vi "AMview.vi"() -> ()   [LabVIEW 2014]
uses:
  TypeDefs/Color.ctl
  TypeDefs/CameraEvent.ctl
  TypeDefs/Camera.ctl
  <vilib>/Utility/miscctls.llb/LV3DPointTypeDef.ctl
  <vilib>/Utility/miscctls.llb/LVStringsAndValuesArrayTypeDef_U16.ctl
  TypeDefs/Point3D.ctl
  <vilib>/picture/3D Picture Control/Object/Add Object (no reference).vi
  <vilib>/picture/3D Picture Control/Object/Create Object (name).vi
  <vilib>/xml/Close Reference(Node).vi
  <vilib>/picture/3D Picture Control/NI_3D Picture Control.lvlib
  <vilib>/xml/NI_XML.lvlib
  <resource>/objmgr/DOMUserDefRef.rc
panel:
  in  "stop":bool
  in  "Toolbar":T1(tab)
  in  "Load":bool
  in  "Line Width":dbl=1.0
  in  "Color Off":T2={"Alpha"=1.0, "Color"=0} {"Alpha" min=0.0 max=1.0 scale=0.0..1.0}
  in  "Line Color":u32(colorbox)=6618880
  in  "Reset":bool
  in  "Ports":enum16{"One Viewport", "Four Viewports"}(ring)
  in  "Build Plate Color":u32(colorbox)=6618880
  in  "Color On":T2={"Alpha"=1.0, "Color"=0} {"Alpha" min=0.0 max=1.0 scale=0.0..1.0}
  in  "Scale":bool
  in  "Percent":dbl=50.0 min=1.0 max=200.0
  in  "ZT":dbl=1.0
  in  "ZPT":bool
  in  "ZNT":bool
  in  "YT":dbl=1.0
  in  "YPT":bool
  in  "YNT":bool
  in  "XT":dbl=1.0
  in  "XPT":bool
  in  "XNT":bool
  in  "Zcen":dbl
  in  "Ycen":dbl
  in  "Xcen":dbl
  in  "Zmax":dbl
  in  "Zmin":dbl
  in  "Ymax":dbl
  in  "Ymin":dbl
  in  "Xmax":dbl
  in  "Xmin":dbl
  in  "ZR":dbl=90.0
  in  "ZRR":bool
  in  "ZLR":bool
  in  "YR":dbl=90.0
  in  "YRR":bool
  in  "YLR":bool
  in  "XR":dbl=90.0
  in  "XRR":bool
  in  "XLR":bool
  in  "Model Selector":u16(ring) items=["GE_SnapBlock_18x9_Repaired"]
  in  "Model Color":T2={"Alpha"=1.0, "Color"=0} {"Alpha" min=0.0 max=1.0 scale=0.0..1.0}
  in  "Layer Thickness":dbl=1.0
  in  "Beam Size":dbl=1.0
  in  "Build Size":dbl=100.0
  in  "SavePath":bool
  in  "Slice":bool
  in  "Z":dbl
  in  "SaveXML":bool
  in  "GenLayer":bool
  out "XML":string
  # "X-->"
  # "Translation"
  # "Scale/Sym"
  # "Rotation"
  # "Bounds"
  # "Y-->"
  # "Z-->"
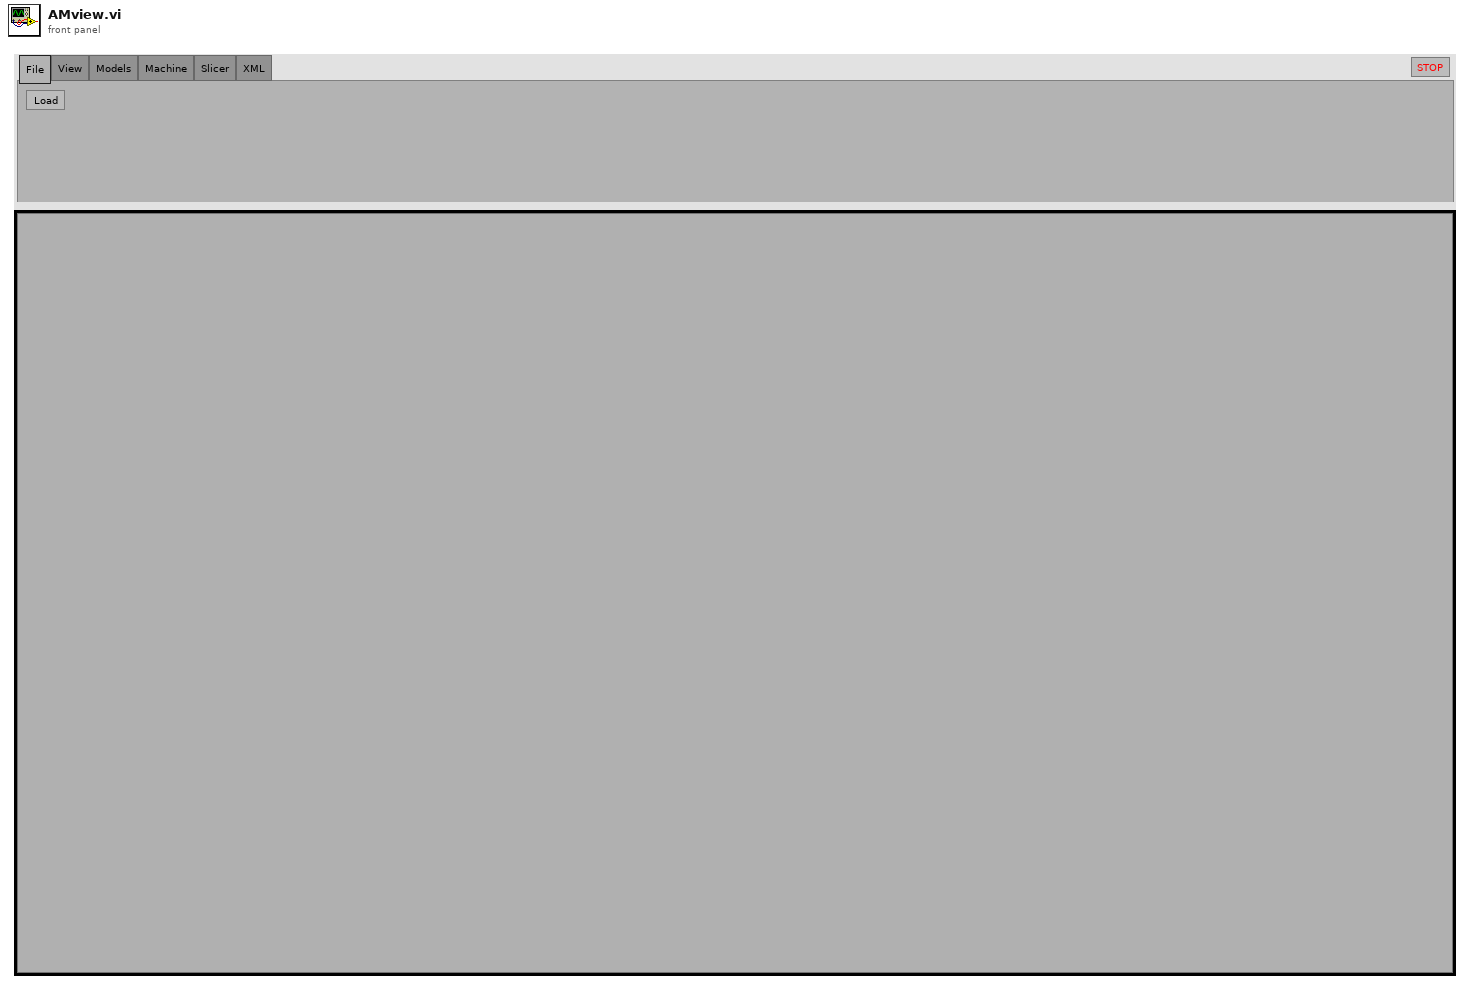
[diagram p1: front panel]
types:
  T1 = enum32{"File", "View", "Models", "Machine", "Slicer", "XML"}
  T2 = typedef "Color.ctl" = cluster{"Alpha":dbl, "Color":u32}
  T3 = enum16{"Add", "Get", "Scale", "Rotate", "Translate", "Symmetry", "Clear"}
  T4 = enum16{"New", "Find", "FindPattern", "GetTable", "Clear"}
  T5 = typedef "LVStringsAndValuesArrayTypeDef_U16.ctl" = cluster{"String":string, "Value":u16}[]
  T6 = typedef "CameraEvent.ctl" = cluster{"Camera":T7, "Task":enum16{"redraw", "setTo", "setToUpdate"}}
  T7 = typedef "Camera.ctl" = cluster{"Camera Position":T8, "Target":T8, "Up Direction":T8}
  T8 = typedef "LV3DPointTypeDef.ctl" = cluster{"X":sgl, "Y":sgl, "Z":sgl}
  T9 = enum16{"Add", "Get", "Scale", "Rotate", "Translate", "Symmetry"}
  T10 = enum16{"Overall", "Per Primitive", "Per Vertex", "Binding Off"}
  T11 = enum16{"Points", "Lines", "Line Strip", "Line Loop", "Triangles", "Triangle Strip", "Triangle Fan", "Quads", "Quad Strip", "Polygon"}
  T12 = cluster{"Axis":enum16{"X", "Y", "Z"}, "Angle":sgl}
  T13 = typedef "Point3D.ctl" = cluster{"X":sgl, "Y":sgl, "Z":sgl}
  T14 = typedef "TriangleFace.ctl" = cluster{"Normal":T13, "Vertex1":T13, "Vertex2":T13, "Vertex3":T13}
  T15 = typedef "Line2D.ctl" = cluster{"Vertex1":T16, "Vertex2":T16, "Slope":dbl}
  T16 = typedef "Point2DwSlope.ctl" = cluster{"X":sgl, "Y":sgl, "Slope":dbl}
  T17 = typedef "Poly2DwSlope.ctl" = cluster{"VertexArray":T16[]}
  T18 = cluster{"VertexArray":T16[], "OnOffAr":enum16{"On", "Off"}[]}
  T19 = cluster{"VertexArray":T16[], enum16{"On", "Off"}[]}
  T20 = cluster{"VertexArray":T16[], "OnOffAr":enum16{"On", "Off"}[]}[]
  T21 = typedef "XYonOffArray.ctl" = cluster{"X":dbl, "Y":dbl, "OnOff":bool}[]
  T22 = typedef "LVRGBAColorTypeDef.ctl" = cluster{"Red":sgl, "Green":sgl, "Blue":sgl, "Alpha":sgl}
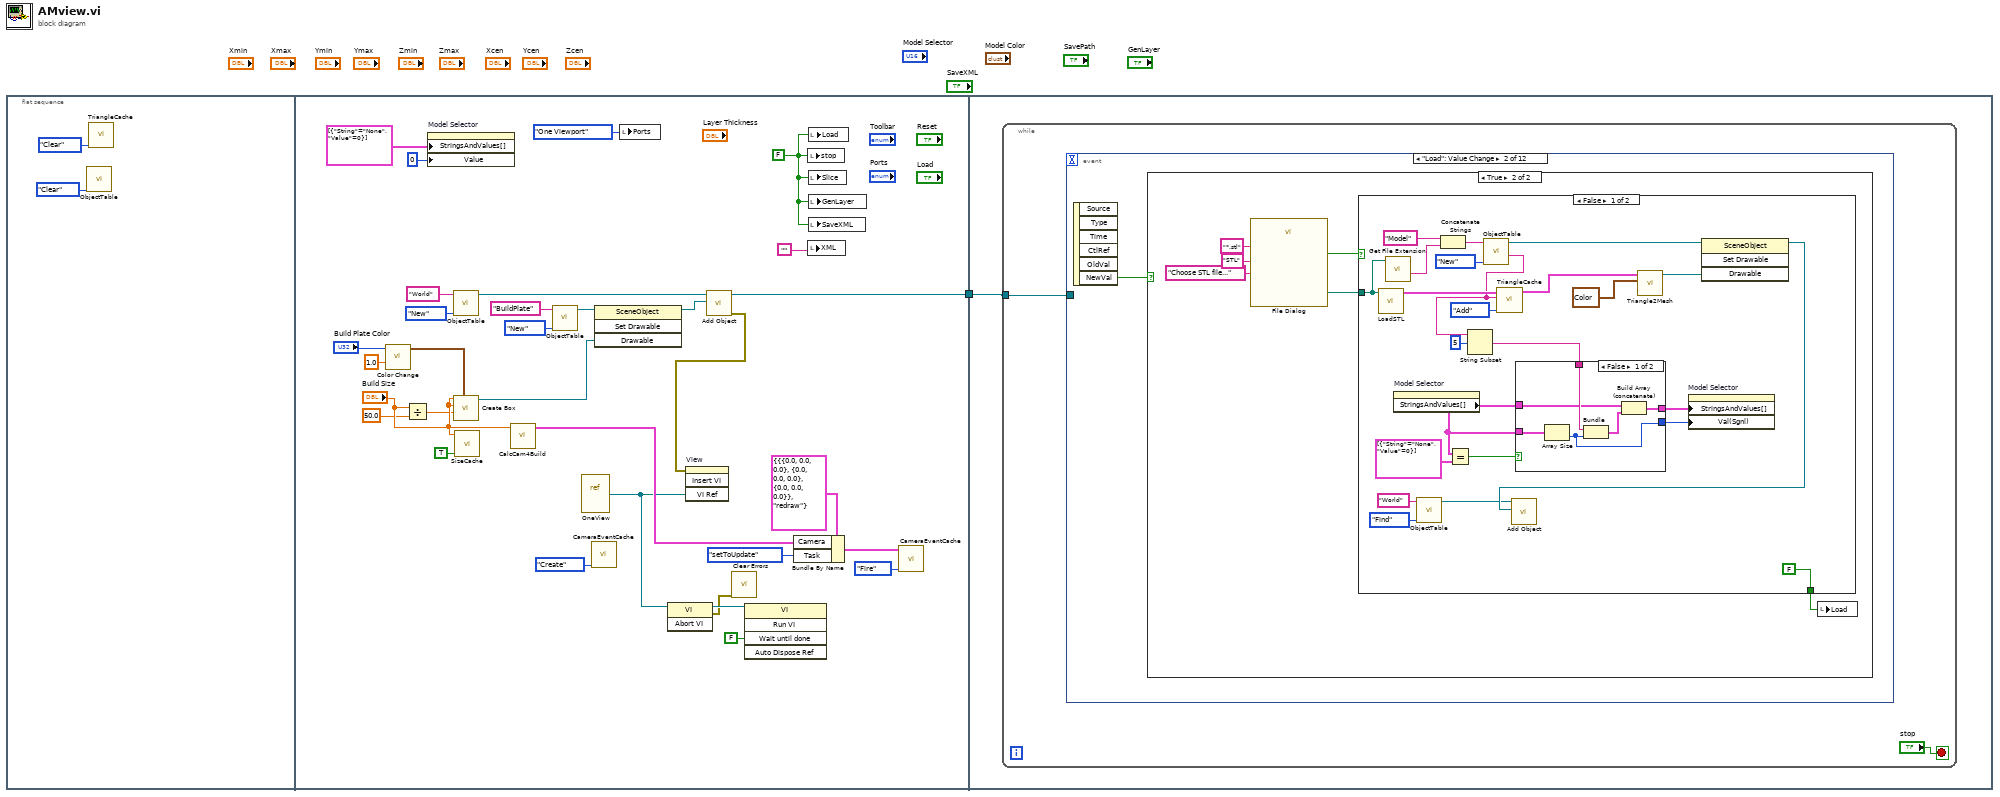
[diagram p0: block diagram]
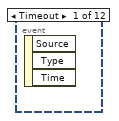
[diagram p2: hidden frame]
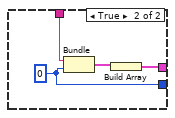
[diagram p4: hidden frame]
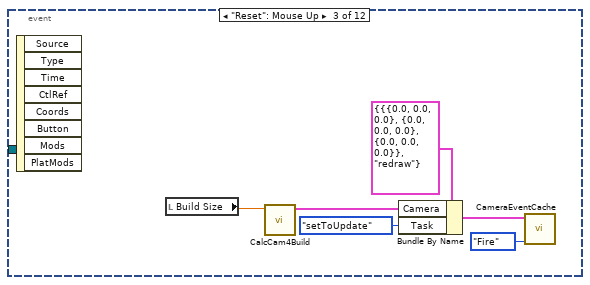
[diagram p6: hidden frame]
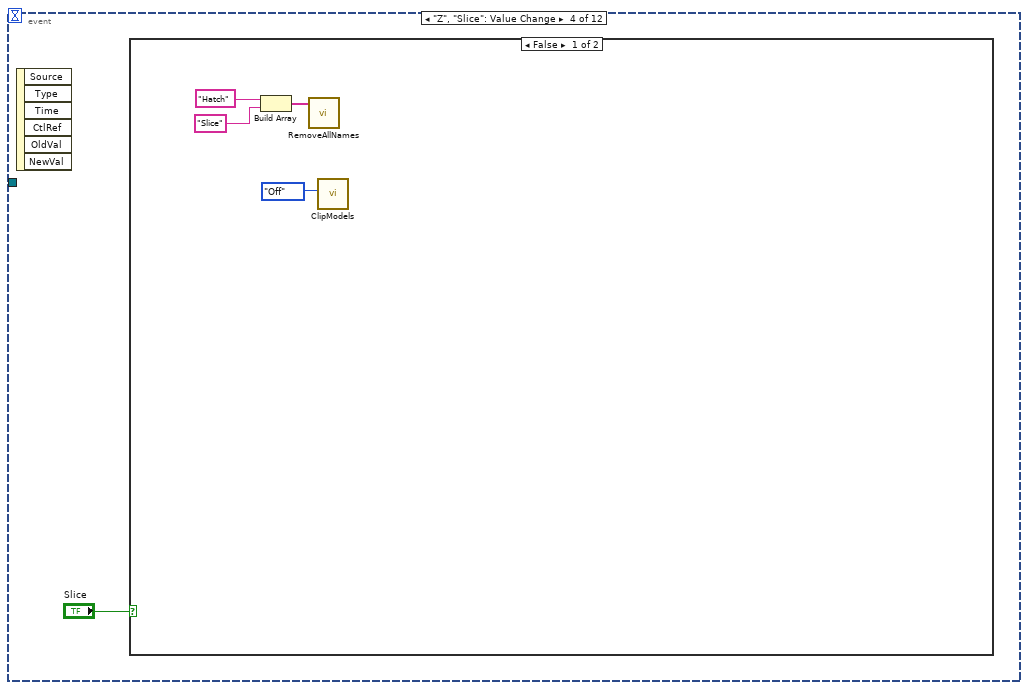
[diagram p7: hidden frame]
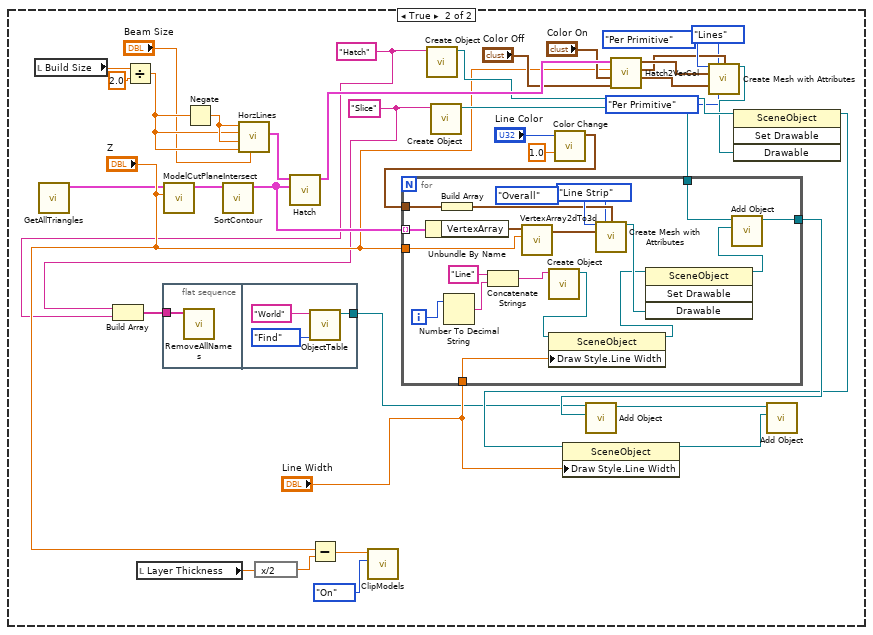
[diagram p8: hidden frame]
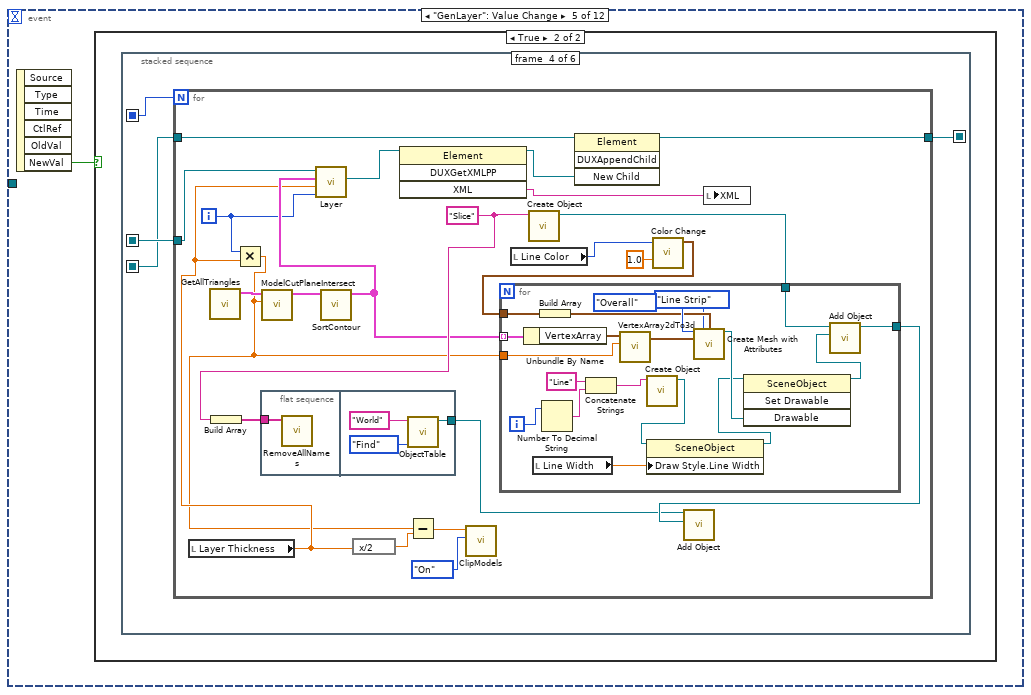
[diagram p9: hidden frame]
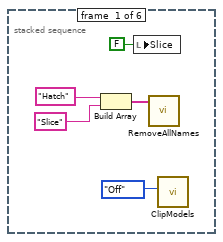
[diagram p11: hidden frame]
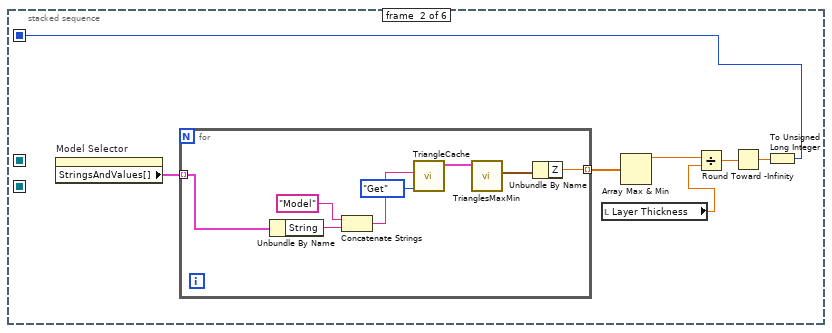
[diagram p12: hidden frame]
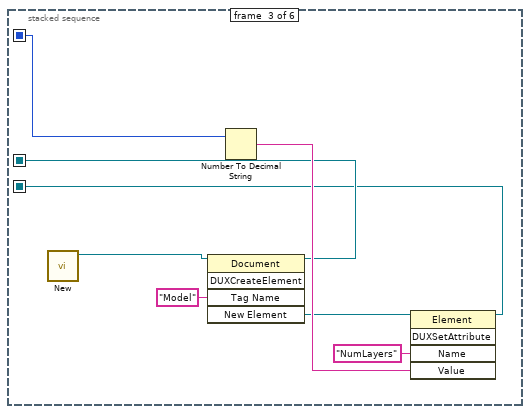
[diagram p13: hidden frame]
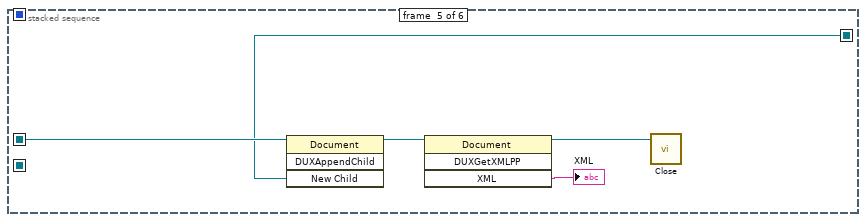
[diagram p14: hidden frame]
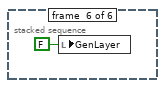
[diagram p15: hidden frame]
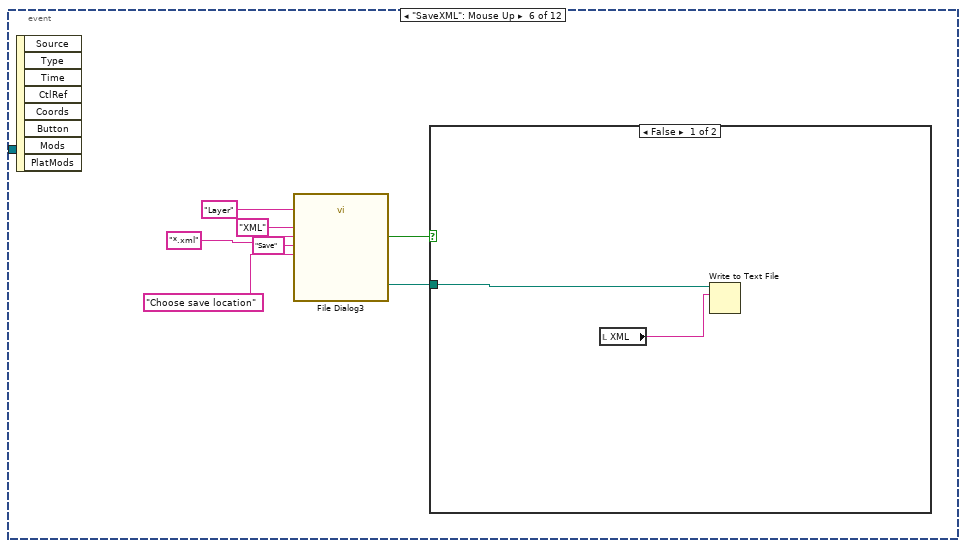
[diagram p16: hidden frame]
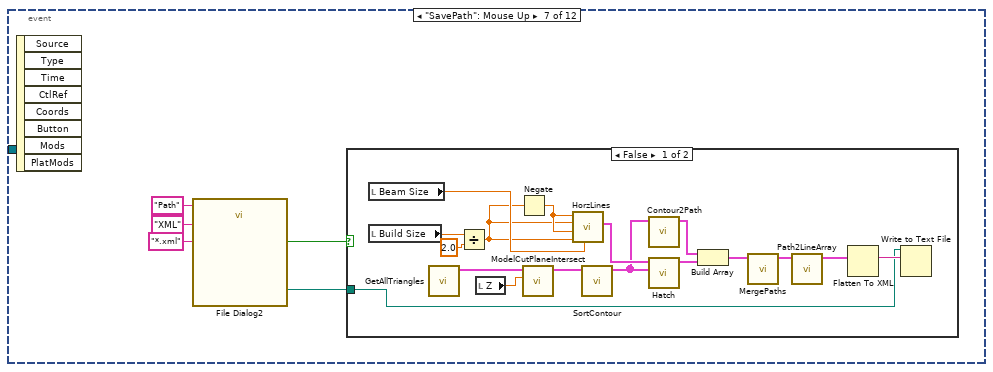
[diagram p18: hidden frame]
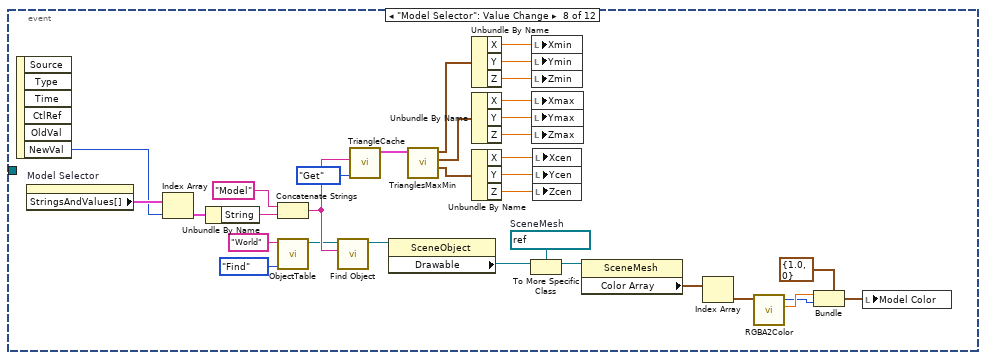
[diagram p20: hidden frame]
diagram:
  n1 = flat-sequence {
    tunnel: [w13] -> w1
    tunnel: w1 -> [w36]
    frame #0 {
      n2 = call "ObjectTable.vi"("ObjectStoreSelector"=T4."Clear") -> ()  [unwired: 6 in, 5 out]
      n3 = call "TriangleCache.vi"("TriangleOperations"=T3."Clear") -> ()  [unwired: 10 in, 1 out]
    }
    frame #1 {
      w5 = FALSE ("stop")
      n4 = call <vilib>:"Color Change.vi"("Alpha"=1.0, "Color"="Build Plate Color") -> ("RGBA"=w17:cluster{"R":sgl, "G":sgl, "B":sgl, "A":sgl})  [unwired: 9 in]
      n5 = Divide(x="Build Size", y=50.0) -> (x/y=w15:dbl)
      n6 = property on="Model Selector" class="Ring (strict)"("StringsAndValues[]"=T5 [{"String"="None", "Value"=0}] ("Strings And Values []"), "Value"=0) -> ()  [unwired: 2 in, 2 out]
      n7 = call "ObjectTable.vi"("ObjectStoreSelector"=enum16{"New", "Find", "FindPattern", "GetTable"}."New", "Name"="World") -> ("ObjectRef"=w31:refnum<vi>)  [unwired: 5 in, 4 out]
      n8 = call <vilib>:"Create Box.vi"("Color"=w17, "Length Z"=w15, "Length Y"="Build Size", "Length X"="Build Size") -> ("New Box Refnum"=w19:refnum<vi>)  [unwired: 6 in, 1 out]
      n9 = call "SizeCache.vi"("Set"=TRUE, "SizeIn"="Build Size") -> ()  [unwired: 9 in, 1 out]
      n10 = call "CalcCam4Build.vi"("BuildSize"="Build Size") -> ("CamOut"=w25:T7)  [unwired: 10 in]
      n11 = call "ObjectTable.vi"("ObjectStoreSelector"=enum16{"New", "Find", "FindPattern", "GetTable"}."New", "Name"="BuildPlate") -> ("ObjectRef"=w33:refnum<vi>)  [unwired: 5 in, 4 out]
      n12 = vi-ref "OneView.vi"() -> (w9:refnum<vi>)
      n13 = call "CameraEventCache.vi"("Operation"=enum16{"Create", "GetRef", "Fire"}."Create") -> ()  [unwired: 10 in, 1 out]
      n14 = invoke class="SceneObject" method="Set Drawable"(reference=w33, "Drawable"=w19) -> (reference out=w20:refnum<vi>)  [unwired: 2 in, 3 out]
      n15 = local write "Ports"(enum16{"One Viewport", "Four Viewports"}."One Viewport" ("Ports")) -> ()
      n16 = invoke class="VI" method="Abort VI"(reference=w9) -> (reference out=w10:refnum<vi>, error out=w6:errorcluster)  [unwired: 2 in, 1 out]
      n17 = call-poly <vilib>:"Add Object.vi"("New Object In"=w20, "Scene Object In"=w31) -> ("error out"=w35:errorcluster, "Scene Object Out"=w13:refnum<vi>)  [unwired: 8 in]
      n18 = invoke on="View" class="SubPanel" method="Insert VI"(error in=w35, "VI Ref"=w9) -> ()  [unwired: 2 in, 4 out]
      n19 = call <vilib>:"Clear Errors.vi"("error in (no error)"=w6) -> ()  [unwired: 5 in, 2 out]
      n20 = invoke class="VI" method="Run VI"(reference=w10, "Wait until done"=FALSE ("Wait Until Done")) -> ()  [unwired: 3 in, 5 out]
      n21 = Bundle By Name(cluster=T6 {"Camera"={"Camera Position"={"X"=0.0, "Y"=0.0, "Z"=0.0}, "Target"={"X"=0.0, "Y"=0.0, "Z"=0.0}, "Up Direction"={"X"=0.0, "Y"=0.0, "Z"=0.0}}, "Task"=enum."redraw"} ("CameraEvent"), "Camera"=w25, "Task"=enum16{"redraw", "setTo", "setToUpdate"}."setToUpdate") -> (w24:T6)
      n22 = local write "stop"(w5) -> ()
      n23 = local write "XML"("") -> ()
      n24 = local write "Load"(w5) -> ()
      n25 = local write "Slice"(w5) -> ()
      n26 = local write "GenLayer"(w5) -> ()
      n27 = local write "SaveXML"(w5) -> ()
      n28 = call "CameraEventCache.vi"("Operation"=enum16{"Create", "GetRef", "Fire"}."Fire", "CameraEvent"=w24) -> ()  [unwired: 9 in, 1 out]
    }
    frame #2 {
      n29 = while {
        tunnel: w36 -> [w37]
        stop <- "stop" stop-if-true
        n30 = event shown="[1] \"Load\": Value Change" {
          selector: _ -> [_ _ _ _ _ _ _ _ _ _ _ _]
          dyn-events: _ -> [_ _ _ _ _ _ _ _ _ _ _ _]
          timeout: _ -> [_ _ _ _ _ _ _ _ _ _ _ _]
          tunnel: w37 -> [_ _ _ _ _ _ _ _ _ _ _ _]
          event Timeout {
            n31 = event-data() -> ()  [unwired: 1 in, 3 out]
          }
          event "Load": Value Change {
            n32 = event-data() -> ("NewVal"=w39:bool)  [unwired: 1 in, 5 out]
            n33 = case shown="True" w39 {
              frame False {
              }
              frame True {
                n34 = call "File Dialog"("prompt"="Choose STL file...", "pattern (all files)"="*.stl", "pattern label"="STL") -> ("selected path"=w41:path, "cancelled"=w42:bool)  [unwired: 9 in, 2 out]
                n35 = case shown="False" w42 {
                  tunnel: w41 -> [w54 _]
                  tunnel: [FALSE _] -> w40
                  frame False {
                    n36 = call "LoadSTL.vi"("STL Path"=w54) -> ("Triangles"=w59:T14[])  [unwired: 8 in, 2 out]
                    n37 = call <vilib>:"Get File Extension.vi"("file"=w54) -> ("filename without extension"=w53:string)  [unwired: 7 in, 3 out]
                    n38 = property on="Model Selector" class="Ring (strict)"() -> ("StringsAndValues[]"=w48:T5)  [unwired: 2 in, 2 out]
                    n39 = call "ObjectTable.vi"("ObjectStoreSelector"=enum16{"New", "Find", "FindPattern", "GetTable"}."Find", "Name"="World") -> ("ObjectRef"=w63:refnum<vi>)  [unwired: 5 in, 4 out]
                    n40 = Concatenate Strings("Model" ("Name"), w53) -> (w66:string)
                    n41 = Equal?(x=w48, y=T5 [{"String"="None", "Value"=0}] ("Strings And Values []")) -> (x = y?=w47:bool)
                    n42 = call "ObjectTable.vi"("ObjectStoreSelector"=enum16{"New", "Find", "FindPattern", "GetTable"}."New", "Name"=w66) -> ("UniqueName"=w51:string, "ObjectRef"=w64:refnum<vi>)  [unwired: 5 in, 3 out]
                    n43 = String Subset(string=w51, offset (0)=5) -> (substring=w52:string)  [unwired: 1 in]
                    n44 = call "TriangleCache.vi"("TriangleOperations"=T9."Add", "ModelName"=w51, "TrianglesIn"=w59) -> ("TrianglesOut"=w58:T14[])  [unwired: 8 in]
                    n45 = case shown="False" w47 {
                      tunnel: [w74 w77] -> w56
                      tunnel: [w73 w76] -> w55
                      tunnel: w52 -> [w72 w79]
                      tunnel: w48 -> [w71 _]
                      tunnel: w48 -> [w70 _]
                      frame False {
                        n46 = Array Size(array=w70) -> (size(s)=w73:i32)
                        n47 = Bundle("UniqueName"=w72, w73) -> (w75:cluster{"UniqueName":string, i32})  [unwired: 1 in]
                        n48 = Build Array (concatenate)(w71, w75) -> (w74:cluster{"UniqueName":string, "Value":i32}[])
                      }
                      frame True {
                        w76 = 0
                        n49 = Bundle("UniqueName"=w79, w76) -> (w78:cluster{"UniqueName":string, i32})  [unwired: 1 in]
                        n50 = Build Array(w78) -> (w77:cluster{"UniqueName":string, i32}[])
                      }
                    }
                    n51 = call "Triangle2Mesh.vi"("Color"=T2 {"Alpha"=1.0, "Color"=16711680}, "Triangles"=w58) -> ("Refnum"=w60:refnum<vi>)  [unwired: 9 in]
                    n52 = property on="Model Selector" class="Ring (strict)"("StringsAndValues[]"=w56, "Val(Sgnl)"=w55) -> ()  [unwired: 2 in, 2 out]
                    n53 = invoke class="SceneObject" method="Set Drawable"(reference=w64, "Drawable"=w60) -> (reference out=w69:refnum<vi>)  [unwired: 2 in, 3 out]
                    n54 = call-poly <vilib>:"Add Object.vi"("New Object In"=w69, "Scene Object In"=w63) -> ()  [unwired: 8 in, 2 out]
                  }
                  frame True {
                  }
                }
                n55 = local write "Load"(w40) -> ()
              }
            }
          }
          event "Reset": Mouse Up {
            n56 = event-data() -> ()  [unwired: 1 in, 8 out]
            n57 = local read "Build Size"() -> (w82:dbl)
            n58 = call "CalcCam4Build.vi"("BuildSize"=w82) -> ("CamOut"=w83:T7)  [unwired: 10 in]
            n59 = Bundle By Name(cluster=T6 {"Camera"={"Camera Position"={"X"=0.0, "Y"=0.0, "Z"=0.0}, "Target"={"X"=0.0, "Y"=0.0, "Z"=0.0}, "Up Direction"={"X"=0.0, "Y"=0.0, "Z"=0.0}}, "Task"=enum."redraw"} ("CameraEvent"), "Camera"=w83, "Task"=enum16{"redraw", "setTo", "setToUpdate"}."setToUpdate") -> (w81:T6)
            n60 = call "CameraEventCache.vi"("Operation"=enum16{"Create", "GetRef", "Fire"}."Fire", "CameraEvent"=w81) -> ()  [unwired: 9 in, 1 out]
          }
          event "Z", "Slice": Value Change {
            n61 = event-data() -> ()  [unwired: 1 in, 6 out]
            n62 = case shown="False" "Slice" {
              frame False {
                n63 = Build Array("Hatch", "Slice") -> (w89:string[])
                n64 = call "RemoveAllNames.vi"("Names"=w89) -> ()  [unwired: 11 in]
                n65 = call "ClipModels.vi"("Clip Plane State"=enum16{"Inherit Value", "Off", "On"}."Off") -> ()  [unwired: 11 in]
              }
              frame True {
                w93 = "Hatch" ("Name")
                w94 = "Slice" ("Name")
                n66 = local read "Build Size"() -> (w126:dbl)
                n67 = call "GetAllTriangles.vi"() -> ("AllTriangles"=w97:T14[])  [unwired: 11 in]
                n68 = Build Array(w94, w93) -> (w92:string[])
                n69 = Divide(x=w126, y=2.0) -> (x/y=w123:dbl)
                n70 = local read "Layer Thickness"() -> (w99:dbl)
                n71 = flat-sequence {
                  tunnel: w92 -> [w129]
                  tunnel: [w130] -> w91
                  frame #0 {
                    n72 = call "RemoveAllNames.vi"("Names"=w129) -> ()  [unwired: 11 in]
                  }
                  frame #1 {
                    n73 = call "ObjectTable.vi"("ObjectStoreSelector"=T4."Find", "Name"="World") -> ("ObjectRef"=w130:refnum<vi>)  [unwired: 5 in, 4 out]
                  }
                }
                n74 = call "ModelCutPlaneIntersect.vi"("CuttingZ"="Z", "Triangles"=w97) -> ("LineArray"=w128:T15[])  [unwired: 8 in, 1 out]
                n75 = Negate(x=w123) -> (-x=w124:dbl)
                n76 = call "SortContour.vi"("LineArray"=w128) -> ("Polys"=w122:T17[])  [unwired: 10 in]
                n77 = call "HorzLines.vi"("Spacing"="Beam Size", "yMax"=w123, "yMin"=w124, "xMax"=w123, "xMin"=w124) -> ("Poly2D"=w127:T17)  [unwired: 5 in, 1 out]
                n78 = expression code="x/2"(w99) -> (w98:dbl)
                n79 = call "Hatch.vi"("Polys"=w122, "Hatch"=w127) -> ("Path"=w116:T18)  [unwired: 9 in]
                n80 = Subtract(x="Z", y=w98) -> (x-y=w96:dbl)
                n81 = call "ClipModels.vi"("Clip Plane State"=enum16{"Inherit Value", "Off", "On"}."On", "Z"=w96) -> ()  [unwired: 10 in]
                n82 = call-poly <vilib>:"Create Object.vi"("Name"=w93) -> ("Scene:New Object"=w109:refnum<vi>)  [unwired: 9 in, 1 out]
                n83 = call-poly <vilib>:"Create Object.vi"("Name"=w94) -> ("Scene:New Object"=w119:refnum<vi>)  [unwired: 9 in, 1 out]
                n84 = call <vilib>:"Color Change.vi"("Alpha"=1.0, "Color"="Line Color") -> ("RGBA"=w120:cluster{"R":sgl, "G":sgl, "B":sgl, "A":sgl})  [unwired: 9 in]
                n85 = for {
                  tunnel: w122 -> [w150] mode=indexing
                  tunnel: "Z" -> [w148]
                  tunnel: w120 -> [w146]
                  tunnel: w119 -> [w139]
                  tunnel: [w138] -> w118
                  tunnel: "Line Width" -> [w133]
                  i -> [w142]
                  n86 = Unbundle By Name(w150) -> ("VertexArray"=w149:T16[])
                  n87 = Build Array(w146) -> (w145:cluster{"R":sgl, "G":sgl, "B":sgl, "A":sgl}[])
                  n88 = Number To Decimal String(number=w142) -> (decimal integer string=w141:string)  [unwired: 1 in]
                  n89 = Concatenate Strings("Line" ("string"), w141) -> (w140:string)
                  n90 = call "VertexArray2dTo3d.vi"("Z"=w148, "VertexArray2D"=w149) -> ("VertexArray3D"=w147:T13[])  [unwired: 9 in]
                  n91 = call-poly <vilib>:"Create Object.vi"("Name"=w140) -> ("Scene:New Object"=w135:refnum<vi>)  [unwired: 9 in, 1 out]
                  n92 = property class="SceneObject"(reference=w135, "Draw Style.Line Width"=w133) -> (reference out=w134:refnum<vi>)  [unwired: 1 in, 1 out]
                  n93 = call <vilib>:"Create Mesh with Attributes.vi"("Draw Mode"=T11."Line Strip", "Color Binding Mode"=T10."Overall", "Color Array"=w145, "Vertex Array"=w147) -> ("New Mesh Refnum"=w137:refnum<vi>)  [unwired: 10 in, 1 out]
                  n94 = invoke class="SceneObject" method="Set Drawable"(reference=w134, "Drawable"=w137) -> (reference out=w136:refnum<vi>)  [unwired: 2 in, 3 out]
                  n95 = call-poly <vilib>:"Add Object.vi"("New Object In"=w136, "Scene Object In"=w139) -> ("Scene Object Out"=w138:refnum<vi>)  [unwired: 8 in, 1 out]
                }
                n96 = call-poly <vilib>:"Add Object.vi"("New Object In"=w118, "Scene Object In"=w91) -> ("Scene Object Out"=w107:refnum<vi>)  [unwired: 8 in, 1 out]
                n97 = call "Hatch2VerCol.vi"("Color Off"="Color Off", "Color On"="Color On", "Z"="Z", "Path"=w116) -> ("Normals"=w102:T13[], "Colors"=w111:cluster{"R":sgl, "G":sgl, "B":sgl, "A":sgl}[], "VertexArray3d"=w112:T13[])  [unwired: 5 in]
                n98 = call <vilib>:"Create Mesh with Attributes.vi"("Draw Mode"=T11."Lines", "Color Binding Mode"=T10."Per Primitive", "Color Array"=w111, "Vertex Array"=w112, "Normal Array"=w102, "Normal Binding Mode"=T10."Per Primitive") -> ("New Mesh Refnum"=w108:refnum<vi>)  [unwired: 8 in, 1 out]
                n99 = invoke class="SceneObject" method="Set Drawable"(reference=w109, "Drawable"=w108) -> (reference out=w105:refnum<vi>)  [unwired: 2 in, 3 out]
                n100 = property class="SceneObject"(reference=w105, "Draw Style.Line Width"="Line Width") -> (reference out=w103:refnum<vi>)  [unwired: 1 in, 1 out]
                n101 = call-poly <vilib>:"Add Object.vi"("New Object In"=w103, "Scene Object In"=w107) -> ()  [unwired: 8 in, 2 out]
              }
            }
          }
          event "GenLayer": Value Change {
            n102 = event-data() -> ("NewVal"=w152:bool)  [unwired: 1 in, 5 out]
            n103 = case shown="True" w152 {
              frame False {
              }
              frame True {
                n104 = stacked-sequence {
                  seq-local: [_ w158 _ _ _ _] -> [_ _ w175 w184 _ _]
                  seq-local: [_ _ w174 _ _ _] -> [_ _ _ w183 w235 _]
                  seq-local: [_ _ w173 _ _ _] -> [_ _ _ w182 _ _]
                  seq-local: [_ _ _ w181 _ _] -> [_ _ _ _ w234 _]
                  frame #0 {
                    n105 = Build Array("Hatch", "Slice") -> (w155:string[])
                    n106 = local write "Slice"(FALSE ("Slice")) -> ()
                    n107 = call "RemoveAllNames.vi"("Names"=w155) -> ()  [unwired: 11 in]
                    n108 = call "ClipModels.vi"("Clip Plane State"=enum16{"Inherit Value", "Off", "On"}."Off") -> ()  [unwired: 11 in]
                  }
                  frame #1 {
                    n109 = property on="Model Selector" class="Ring (strict)"() -> ("StringsAndValues[]"=w164:T5)  [unwired: 2 in, 2 out]
                    n110 = for {
                      tunnel: w164 -> [w167] mode=indexing
                      tunnel: [w165] -> w163 mode=indexing
                      n111 = Unbundle By Name(w167) -> ("String"=w172:string)
                      n112 = Concatenate Strings("Model" ("string"), w172) -> (w168:string)
                      n113 = call "TriangleCache.vi"("TriangleOperations"=T3."Get", "ModelName"=w168) -> ("TrianglesOut"=w169:T14[])  [unwired: 9 in]
                      n114 = call "TrianglesMaxMin.vi"("Triangles"=w169) -> ("MaxDims"=w166:T13)  [unwired: 8 in, 2 out]
                      n115 = Unbundle By Name(w166) -> ("Z"=w165:sgl)
                    }
                    n116 = local read "Layer Thickness"() -> (w161:dbl)
                    n117 = Array Max & Min(array=w163) -> (max value=w162:sgl)  [unwired: 3 out]
                    n118 = Divide(x=w162, y=w161) -> (x/y=w160:dbl)
                    n119 = Round Toward -Infinity(1:w160) -> (0:w159:dbl)
                    n120 = To Unsigned Long Integer(number=w159) -> (unsigned 32bit integer=w158:u32)
                  }
                  frame #2 {
                    n121 = call <vilib>:"New.vi"() -> ("DOM document out"=w177:refnum<k20>)  [unwired: 8 in, 1 out]
                    n122 = invoke class="Document" method="DUXCreateElement"(reference=w177, "Tag Name"="Model") -> (reference out=w174:refnum<k20>, "New Element"=w176:refnum<k20>)  [unwired: 3 in, 3 out]
                    n123 = Number To Decimal String(number=w175) -> (decimal integer string=w178:string)  [unwired: 1 in]
                    n124 = invoke class="Element" method="DUXSetAttribute"(reference=w176, "Name"="NumLayers", "Value"=w178) -> (reference out=w173:refnum<k20>)  [unwired: 2 in, 4 out]
                  }
                  frame #3 {
                    n125 = for {
                      N: w184 -> [_]
                      tunnel: w183 -> [w194]
                      tunnel: w182 -> [w192]
                      tunnel: [w191] -> w181
                      i -> [w190]
                      w197 = "Slice" ("Name")
                      n126 = local read "Layer Thickness"() -> (w189:dbl)
                      n127 = call "GetAllTriangles.vi"() -> ("AllTriangles"=w200:T14[])  [unwired: 11 in]
                      n128 = Build Array(w197) -> (w196:string[])
                      n129 = Multiply(x=w190, y=w189) -> (x*y=w188:dbl)
                      n130 = flat-sequence {
                        tunnel: w196 -> [w208]
                        tunnel: [w209] -> w195
                        frame #0 {
                          n131 = call "RemoveAllNames.vi"("Names"=w208) -> ()  [unwired: 11 in]
                        }
                        frame #1 {
                          n132 = call "ObjectTable.vi"("ObjectStoreSelector"=T4."Find", "Name"="World") -> ("ObjectRef"=w209:refnum<vi>)  [unwired: 5 in, 4 out]
                        }
                      }
                      n133 = call "ModelCutPlaneIntersect.vi"("CuttingZ"=w188, "Triangles"=w200) -> ("LineArray"=w206:T15[])  [unwired: 8 in, 1 out]
                      n134 = call "SortContour.vi"("LineArray"=w206) -> ("Polys"=w193:T17[])  [unwired: 10 in]
                      n135 = call "Layer.vi"("Index"=w190, "Thickness"=w189, "Contours"=w193, "DocIn"=w194) -> ("Layer"=w187:refnum<k20>)  [unwired: 6 in, 1 out]
                      n136 = expression code="x/2"(w189) -> (w201:dbl)
                      n137 = invoke class="Element" method="DUXGetXMLPP"(reference=w187) -> (reference out=w186:refnum<k20>, "XML"=w185:string)  [unwired: 3 in, 2 out]
                      n138 = Subtract(x=w188, y=w201) -> (x-y=w199:dbl)
                      n139 = call "ClipModels.vi"("Clip Plane State"=enum16{"Inherit Value", "Off", "On"}."On", "Z"=w199) -> ()  [unwired: 10 in]
                      n140 = local read "Line Color"() -> (w207:u32)
                      n141 = call-poly <vilib>:"Create Object.vi"("Name"=w197) -> ("Scene:New Object"=w204:refnum<vi>)  [unwired: 9 in, 1 out]
                      n142 = invoke class="Element" method="DUXAppendChild"(reference=w192, "New Child"=w186) -> (reference out=w191:refnum<k20>)  [unwired: 2 in, 3 out]
                      n143 = call <vilib>:"Color Change.vi"("Alpha"=1.0, "Color"=w207) -> ("RGBA"=w205:cluster{"R":sgl, "G":sgl, "B":sgl, "A":sgl})  [unwired: 9 in]
                      n144 = for {
                        tunnel: w193 -> [w229] mode=indexing
                        tunnel: w188 -> [w227]
                        tunnel: w205 -> [w225]
                        tunnel: w204 -> [w218]
                        tunnel: [w217] -> w203
                        i -> [w221]
                        n145 = Unbundle By Name(w229) -> ("VertexArray"=w228:T16[])
                        n146 = local read "Line Width"() -> (w212:dbl)
                        n147 = Build Array(w225) -> (w224:cluster{"R":sgl, "G":sgl, "B":sgl, "A":sgl}[])
                        n148 = Number To Decimal String(number=w221) -> (decimal integer string=w220:string)  [unwired: 1 in]
                        n149 = Concatenate Strings("Line" ("string"), w220) -> (w219:string)
                        n150 = call "VertexArray2dTo3d.vi"("Z"=w227, "VertexArray2D"=w228) -> ("VertexArray3D"=w226:T13[])  [unwired: 9 in]
                        n151 = call-poly <vilib>:"Create Object.vi"("Name"=w219) -> ("Scene:New Object"=w214:refnum<vi>)  [unwired: 9 in, 1 out]
                        n152 = property class="SceneObject"(reference=w214, "Draw Style.Line Width"=w212) -> (reference out=w213:refnum<vi>)  [unwired: 1 in, 1 out]
                        n153 = call <vilib>:"Create Mesh with Attributes.vi"("Draw Mode"=T11."Line Strip", "Color Binding Mode"=T10."Overall", "Color Array"=w224, "Vertex Array"=w226) -> ("New Mesh Refnum"=w216:refnum<vi>)  [unwired: 10 in, 1 out]
                        n154 = invoke class="SceneObject" method="Set Drawable"(reference=w213, "Drawable"=w216) -> (reference out=w215:refnum<vi>)  [unwired: 2 in, 3 out]
                        n155 = call-poly <vilib>:"Add Object.vi"("New Object In"=w215, "Scene Object In"=w218) -> ("Scene Object Out"=w217:refnum<vi>)  [unwired: 8 in, 1 out]
                      }
                      n156 = call-poly <vilib>:"Add Object.vi"("New Object In"=w203, "Scene Object In"=w195) -> ()  [unwired: 8 in, 2 out]
                      n157 = local write "XML"(w185) -> ()
                    }
                  }
                  frame #4 {
                    n158 = invoke class="Document" method="DUXAppendChild"(reference=w235, "New Child"=w234) -> (reference out=w233:refnum<k20>)  [unwired: 2 in, 3 out]
                    n159 = invoke class="Document" method="DUXGetXMLPP"(reference=w233) -> (reference out=w231:refnum<k20>, "XML"=→"XML":string)  [unwired: 3 in, 2 out]
                    n160 = call-poly <vilib>:"Close.vi"("node"=w231) -> ()  [unwired: 8 in, 1 out]
                  }
                  frame #5 {
                    n161 = local write "GenLayer"(FALSE ("GenLayer")) -> ()
                  }
                }
              }
            }
          }
          event "SaveXML": Mouse Up {
            n162 = event-data() -> ()  [unwired: 1 in, 8 out]
            n163 = call "File Dialog3"("prompt"="Choose save location", "button label"="Save", "default name"="Layer", "pattern (all files)"="XML", "pattern label"="*.xml") -> ("selected path"=w237:path, "cancelled"=w238:bool)  [unwired: 7 in, 2 out]
            n164 = case shown="False" w238 {
              tunnel: w237 -> [w244 _]
              frame False {
                n165 = local read "XML"() -> (w245:string)
                n166 = Write to Text File(file (use dialog)=w244, text=w245) -> ()  [unwired: 2 in, 3 out]
              }
              frame True {
              }
            }
          }
          event "SavePath": Mouse Up {
            n167 = event-data() -> ()  [unwired: 1 in, 8 out]
            n168 = call "File Dialog2"("default name"="Path", "pattern (all files)"="XML", "pattern label"="*.xml") -> ("selected path"=w246:path, "cancelled"=w247:bool)  [unwired: 9 in, 2 out]
            n169 = case shown="False" w247 {
              tunnel: w246 -> [w256 _]
              frame False {
                n170 = local read "Beam Size"() -> (w266:dbl)
                n171 = local read "Build Size"() -> (w263:dbl)
                n172 = call "GetAllTriangles.vi"() -> ("AllTriangles"=w259:T14[])  [unwired: 11 in]
                n173 = Divide(x=w263, y=2.0) -> (x/y=w260:dbl)
                n174 = local read "Z"() -> (w267:dbl)
                n175 = Negate(x=w260) -> (-x=w261:dbl)
                n176 = call "ModelCutPlaneIntersect.vi"("CuttingZ"=w267, "Triangles"=w259) -> ("LineArray"=w265:T15[])  [unwired: 8 in, 1 out]
                n177 = call "HorzLines.vi"("Spacing"=w266, "yMax"=w260, "yMin"=w261, "xMax"=w260, "xMin"=w261) -> ("Poly2D"=w264:T17)  [unwired: 5 in, 1 out]
                n178 = call "SortContour.vi"("LineArray"=w265) -> ("Polys"=w255:T17[])  [unwired: 10 in]
                n179 = call "Contour2Path.vi"("Polys"=w255) -> ("Path"=w253:T19)  [unwired: 10 in]
                n180 = call "Hatch.vi"("Polys"=w255, "Hatch"=w264) -> ("Path"=w254:T18)  [unwired: 9 in]
                n181 = Build Array(w253, w254) -> (w251:T20)
                n182 = call "MergePaths.vi"("PathArray"=w251) -> ("PathOut"=w252:T18)  [unwired: 10 in]
                n183 = call "Path2LineArray.vi"("Path"=w252) -> ("LineArray"=w258:T21)  [unwired: 10 in]
                n184 = Flatten To XML(anything=w258) -> (xml string=w257:string)
                n185 = Write to Text File(file (use dialog)=w256, text=w257) -> ()  [unwired: 2 in, 3 out]
              }
              frame True {
              }
            }
          }
          event "Model Selector": Value Change {
            w295 = refnum<vi> refnum  # SceneMesh
            n186 = event-data() -> ("NewVal"=w299:u16)  [unwired: 1 in, 5 out]
            n187 = property on="Model Selector" class="Ring (strict)"() -> ("StringsAndValues[]"=w300:T5)  [unwired: 2 in, 2 out]
            n188 = Index Array(array=w300, index=w299) -> (element=w298:cluster{"String":string, "Value":u16})
            n189 = Unbundle By Name(w298) -> ("String"=w297:string)
            n190 = Concatenate Strings("Model" ("string"), w297) -> (w272:string)
            n191 = call "ObjectTable.vi"("ObjectStoreSelector"=T4."Find", "Name"="World") -> ("ObjectRef"=w269:refnum<vi>)  [unwired: 5 in, 4 out]
            n192 = call <vilib>:"Find Object.vi"("Object Name"=w272, "Scene Refnum"=w269) -> ("Object Refnum"=w268:refnum<vi>)  [unwired: 8 in, 1 out]
            n193 = call "TriangleCache.vi"("TriangleOperations"=T3."Get", "ModelName"=w272) -> ("TrianglesOut"=w286:T14[])  [unwired: 9 in]
            n194 = property class="SceneObject"(reference=w268) -> ("Drawable"=w273:refnum<vi>)  [unwired: 1 in, 2 out]
            n195 = call "TrianglesMaxMin.vi"("Triangles"=w286) -> ("Center"=w283:T13, "MaxDims"=w284:T13, "MinDims"=w285:T13)  [unwired: 8 in]
            n196 = Unbundle By Name(w285) -> ("X"=w282:sgl, "Y"=w281:sgl, "Z"=w280:sgl)
            n197 = Unbundle By Name(w284) -> ("X"=w279:sgl, "Y"=w278:sgl, "Z"=w277:sgl)
            n198 = Unbundle By Name(w283) -> ("X"=w276:sgl, "Y"=w275:sgl, "Z"=w274:sgl)
            n199 = To More Specific Class(target class=w295, reference=w273) -> (specific class reference=w294:refnum<vi>)  [unwired: 1 in, 1 out]
            n200 = local write "Xmin"(w282) -> ()
            n201 = local write "Ymin"(w281) -> ()
            n202 = local write "Zmin"(w280) -> ()
            n203 = local write "Xmax"(w279) -> ()
            n204 = local write "Ymax"(w278) -> ()
            n205 = local write "Zmax"(w277) -> ()
            n206 = local write "Xcen"(w276) -> ()
            n207 = local write "Ycen"(w275) -> ()
            n208 = local write "Zcen"(w274) -> ()
            n209 = property class="SceneMesh"(reference=w294) -> ("Color Array"=w293:T22[])  [unwired: 1 in, 2 out]
            n210 = Index Array(array=w293) -> (element=w292:T22)  [unwired: 1 in]
            n211 = call "RGBA2Color.vi"("RGBA"=w292) -> ("Alpha"=w290:dbl, "Color"=w289:u32)  [unwired: 9 in]
            n212 = Bundle(cluster=T2 {"Alpha"=1.0, "Color"=0} ("Color"), "Alpha"=w290, "Color"=w289) -> (w288:T2)
            n213 = local write "Model Color"(w288) -> ()
          }
          event "XLR", "XRR", "YLR", "YRR", "ZLR", "ZRR": Mouse Up {
            n214 = event-data() -> ("CtlRef"=w325:refnum<vi>)  [unwired: 1 in, 7 out]
            n215 = local read "Model Selector"() -> (w326:u16)
            n216 = property on="Model Selector" class="Ring (strict)"() -> ("StringsAndValues[]"=w333:T5)  [unwired: 2 in, 2 out]
            n217 = property class="Bool (strict)"(reference=w325) -> ("Label.Text"=w324:string)  [unwired: 1 in, 2 out]
            n218 = Index Array(array=w333, index=w326) -> (element=w332:cluster{"String":string, "Value":u16})
            n219 = Unbundle By Name(w332) -> ("String"=w331:string)
            n220 = case shown="\"XLR\", Default" w324 {
              tunnel: T12 {"Axis"=enum."X", "Angle"=0.0} ("Rotation") -> [w337 w342 w346 w351 w355 w360]
              tunnel: "XR" -> [w335 w339 _ _ _ _]
              tunnel: [w334 w340 w344 w349 w353 w358] -> w320
              tunnel: "YR" -> [_ _ w343 w348 _ _]
              tunnel: "ZR" -> [_ _ _ _ w352 w357]
              frame "XLR", Default {
                n221 = Bundle By Name(cluster=w337, "Axis"=enum16{"X", "Y", "Z"}."X", "Angle"=w335) -> (w334:T12)
              }
              frame "XRR" {
                n222 = Negate(x=w339) -> (-x=w338:dbl)
                n223 = Bundle By Name(cluster=w342, "Axis"=enum16{"X", "Y", "Z"}."X", "Angle"=w338) -> (w340:T12)
              }
              frame "YLR" {
                n224 = Bundle By Name(cluster=w346, "Axis"=enum16{"X", "Y", "Z"}."Y", "Angle"=w343) -> (w344:T12)
              }
              frame "YRR" {
                n225 = Negate(x=w348) -> (-x=w347:dbl)
                n226 = Bundle By Name(cluster=w351, "Axis"=enum16{"X", "Y", "Z"}."Y", "Angle"=w347) -> (w349:T12)
              }
              frame "ZLR" {
                n227 = Bundle By Name(cluster=w355, "Axis"=enum16{"X", "Y", "Z"}."Z", "Angle"=w352) -> (w353:T12)
              }
              frame "ZRR" {
                n228 = Negate(x=w357) -> (-x=w356:dbl)
                n229 = Bundle By Name(cluster=w360, "Axis"=enum16{"X", "Y", "Z"}."Z", "Angle"=w356) -> (w358:T12)
              }
            }
            n230 = Concatenate Strings("Model" ("string"), w331) -> (w323:string)
            n231 = call "ObjectTable.vi"("ObjectStoreSelector"=T4."Find", "Name"="World") -> ("ObjectRef"=w327:refnum<vi>)  [unwired: 5 in, 4 out]
            n232 = call <vilib>:"Find Object.vi"("Object Name"=w323, "Scene Refnum"=w327) -> ("Object Refnum"=w318:refnum<vi>)  [unwired: 8 in, 1 out]
            n233 = local read "Model Color"() -> (w317:T2)
            n234 = call "TriangleCache.vi"("Rotation"=w320, "TriangleOperations"=T3."Rotate", "ModelName"=w323) -> ("TrianglesOut"=w301:T14[])  [unwired: 8 in]
            n235 = call "Triangle2Mesh.vi"("Color"=w317, "Triangles"=w301) -> ("Refnum"=w316:refnum<vi>)  [unwired: 9 in]
            n236 = invoke class="SceneObject" method="Set Drawable"(reference=w318, "Drawable"=w316) -> ()  [unwired: 2 in, 4 out]
            n237 = call "TrianglesMaxMin.vi"("Triangles"=w301) -> ("Center"=w311:T13, "MaxDims"=w312:T13, "MinDims"=w313:T13)  [unwired: 8 in]
            n238 = Unbundle By Name(w313) -> ("X"=w310:sgl, "Y"=w309:sgl, "Z"=w308:sgl)
            n239 = Unbundle By Name(w312) -> ("X"=w307:sgl, "Y"=w306:sgl, "Z"=w305:sgl)
            n240 = Unbundle By Name(w311) -> ("X"=w304:sgl, "Y"=w303:sgl, "Z"=w302:sgl)
            n241 = local write "Xmin"(w310) -> ()
            n242 = local write "Ymin"(w309) -> ()
            n243 = local write "Zmin"(w308) -> ()
            n244 = local write "Xmax"(w307) -> ()
            n245 = local write "Ymax"(w306) -> ()
            n246 = local write "Zmax"(w305) -> ()
            n247 = local write "Xcen"(w304) -> ()
            n248 = local write "Ycen"(w303) -> ()
            n249 = local write "Zcen"(w302) -> ()
          }
          event "XNT", "YNT", "ZNT", "XPT", "YPT", "ZPT": Mouse Up {
            n250 = event-data() -> ("CtlRef"=w366:refnum<vi>)  [unwired: 1 in, 7 out]
            n251 = local read "Model Selector"() -> (w386:u16)
            n252 = property on="Model Selector" class="Ring (strict)"() -> ("StringsAndValues[]"=w393:T5)  [unwired: 2 in, 2 out]
            n253 = property class="Bool (strict)"(reference=w366) -> ("Label.Text"=w385:string)  [unwired: 1 in, 2 out]
            n254 = Index Array(array=w393, index=w386) -> (element=w392:cluster{"String":string, "Value":u16})
            n255 = Unbundle By Name(w392) -> ("String"=w391:string)
            n256 = case shown="\"XPT\", Default" w385 {
              tunnel: T13 {"X"=0.0, "Y"=0.0, "Z"=0.0} ("Point3D") -> [w396 w400 w403 w407 w410 w414]
              tunnel: "XT" -> [w395 w398 _ _ _ _]
              tunnel: [w394 w399 w402 w406 w409 w413] -> w362
              tunnel: "YT" -> [_ _ w401 w405 _ _]
              tunnel: "ZT" -> [_ _ _ _ w408 w412]
              frame "XPT", Default {
                n257 = Bundle By Name(cluster=w396, "X"=w395) -> (w394:T13)
              }
              frame "XNT" {
                n258 = Negate(x=w398) -> (-x=w397:dbl)
                n259 = Bundle By Name(cluster=w400, "X"=w397) -> (w399:T13)
              }
              frame "YPT" {
                n260 = Bundle By Name(cluster=w403, "Y"=w401) -> (w402:T13)
              }
              frame "YNT" {
                n261 = Negate(x=w405) -> (-x=w404:dbl)
                n262 = Bundle By Name(cluster=w407, "Y"=w404) -> (w406:T13)
              }
              frame "ZPT" {
                n263 = Bundle By Name(cluster=w410, "Z"=w408) -> (w409:T13)
              }
              frame "ZNT" {
                n264 = Negate(x=w412) -> (-x=w411:dbl)
                n265 = Bundle By Name(cluster=w414, "Z"=w411) -> (w413:T13)
              }
            }
            n266 = Concatenate Strings("Model" ("string"), w391) -> (w384:string)
            n267 = call "ObjectTable.vi"("ObjectStoreSelector"=T4."Find", "Name"="World") -> ("ObjectRef"=w387:refnum<vi>)  [unwired: 5 in, 4 out]
            n268 = call <vilib>:"Find Object.vi"("Object Name"=w384, "Scene Refnum"=w387) -> ("Object Refnum"=w382:refnum<vi>)  [unwired: 8 in, 1 out]
            n269 = local read "Model Color"() -> (w381:T2)
            n270 = call "TriangleCache.vi"("Point3D"=w362, "TriangleOperations"=T3."Translate", "ModelName"=w384) -> ("TrianglesOut"=w367:T14[])  [unwired: 8 in]
            n271 = call "Triangle2Mesh.vi"("Color"=w381, "Triangles"=w367) -> ("Refnum"=w380:refnum<vi>)  [unwired: 9 in]
            n272 = invoke class="SceneObject" method="Set Drawable"(reference=w382, "Drawable"=w380) -> ()  [unwired: 2 in, 4 out]
            n273 = call "TrianglesMaxMin.vi"("Triangles"=w367) -> ("Center"=w377:T13, "MaxDims"=w378:T13, "MinDims"=w379:T13)  [unwired: 8 in]
            n274 = Unbundle By Name(w379) -> ("X"=w376:sgl, "Y"=w375:sgl, "Z"=w374:sgl)
            n275 = Unbundle By Name(w378) -> ("X"=w373:sgl, "Y"=w372:sgl, "Z"=w371:sgl)
            n276 = Unbundle By Name(w377) -> ("X"=w370:sgl, "Y"=w369:sgl, "Z"=w368:sgl)
            n277 = local write "Xmin"(w376) -> ()
            n278 = local write "Ymin"(w375) -> ()
            n279 = local write "Zmin"(w374) -> ()
            n280 = local write "Xmax"(w373) -> ()
            n281 = local write "Ymax"(w372) -> ()
            n282 = local write "Zmax"(w371) -> ()
            n283 = local write "Xcen"(w370) -> ()
            n284 = local write "Ycen"(w369) -> ()
            n285 = local write "Zcen"(w368) -> ()
          }
          event "Scale": Mouse Up {
            n286 = event-data() -> ()  [unwired: 1 in, 8 out]
            n287 = local read "Model Selector"() -> (w435:u16)
            n288 = property on="Model Selector" class="Ring (strict)"() -> ("StringsAndValues[]"=w442:T5)  [unwired: 2 in, 2 out]
            n289 = Index Array(array=w442, index=w435) -> (element=w441:cluster{"String":string, "Value":u16})
            n290 = Unbundle By Name(w441) -> ("String"=w440:string)
            n291 = Concatenate Strings("Model" ("string"), w440) -> (w434:string)
            n292 = call "ObjectTable.vi"("ObjectStoreSelector"=T4."Find", "Name"="World") -> ("ObjectRef"=w436:refnum<vi>)  [unwired: 5 in, 4 out]
            n293 = call <vilib>:"Find Object.vi"("Object Name"=w434, "Scene Refnum"=w436) -> ("Object Refnum"=w432:refnum<vi>)  [unwired: 8 in, 1 out]
            n294 = expression code="x/100"("Percent") -> (w415:dbl)
            n295 = local read "Model Color"() -> (w431:T2)
            n296 = call "TriangleCache.vi"("TriangleOperations"=T3."Scale", "ScaleFac"=w415, "ModelName"=w434) -> ("TrianglesOut"=w417:T14[])  [unwired: 8 in]
            n297 = call "Triangle2Mesh.vi"("Color"=w431, "Triangles"=w417) -> ("Refnum"=w430:refnum<vi>)  [unwired: 9 in]
            n298 = invoke class="SceneObject" method="Set Drawable"(reference=w432, "Drawable"=w430) -> ()  [unwired: 2 in, 4 out]
            n299 = call "TrianglesMaxMin.vi"("Triangles"=w417) -> ("Center"=w427:T13, "MaxDims"=w428:T13, "MinDims"=w429:T13)  [unwired: 8 in]
            n300 = Unbundle By Name(w429) -> ("X"=w426:sgl, "Y"=w425:sgl, "Z"=w424:sgl)
            n301 = Unbundle By Name(w428) -> ("X"=w423:sgl, "Y"=w422:sgl, "Z"=w421:sgl)
            n302 = Unbundle By Name(w427) -> ("X"=w420:sgl, "Y"=w419:sgl, "Z"=w418:sgl)
            n303 = local write "Xmin"(w426) -> ()
            n304 = local write "Ymin"(w425) -> ()
            n305 = local write "Zmin"(w424) -> ()
            n306 = local write "Xmax"(w423) -> ()
            n307 = local write "Ymax"(w422) -> ()
            n308 = local write "Zmax"(w421) -> ()
            n309 = local write "Xcen"(w420) -> ()
            n310 = local write "Ycen"(w419) -> ()
            n311 = local write "Zcen"(w418) -> ()
          }
          event Value Change {
            n312 = event-data() -> ("NewVal"=w443:T2)  [unwired: 1 in, 5 out]
            n313 = local read "Model Selector"() -> (w449:u16)
            n314 = property on="Model Selector" class="Ring (strict)"() -> ("StringsAndValues[]"=w456:T5)  [unwired: 2 in, 2 out]
            n315 = Index Array(array=w456, index=w449) -> (element=w455:cluster{"String":string, "Value":u16})
            n316 = Unbundle By Name(w455) -> ("String"=w454:string)
            n317 = Concatenate Strings("Model" ("string"), w454) -> (w448:string)
            n318 = call "ObjectTable.vi"("ObjectStoreSelector"=T4."Find", "Name"="World") -> ("ObjectRef"=w450:refnum<vi>)  [unwired: 5 in, 4 out]
            n319 = call <vilib>:"Find Object.vi"("Object Name"=w448, "Scene Refnum"=w450) -> ("Object Refnum"=w446:refnum<vi>)  [unwired: 8 in, 1 out]
            n320 = call "TriangleCache.vi"("TriangleOperations"=T3."Get", "ModelName"=w448) -> ("TrianglesOut"=w444:T14[])  [unwired: 9 in]
            n321 = call "Triangle2Mesh.vi"("Color"=w443, "Triangles"=w444) -> ("Refnum"=w445:refnum<vi>)  [unwired: 9 in]
            n322 = invoke class="SceneObject" method="Set Drawable"(reference=w446, "Drawable"=w445) -> ()  [unwired: 2 in, 4 out]
          }
        }
      }
    }
  }
